vi "rename object.vi"(8 "error in":errorcluster, 9 "label_visible":bool, 10 "new_label_name":string, 11 "id":string) -> (0 "error out":errorcluster)   [LabVIEW 2020]
doc: "Renames an objects label.text property, can be a control/indicator or a block diagram element like a constant."
uses:
  G-AI Core/G-AI Core.lvlib
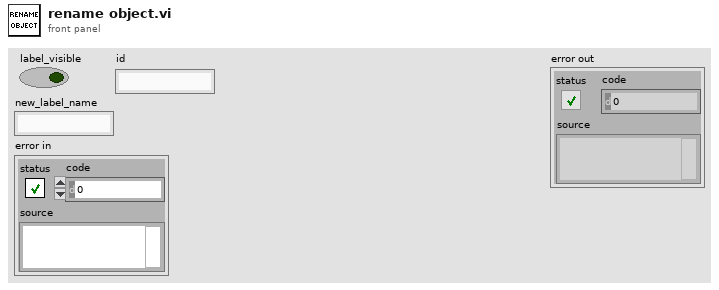
[diagram p1: front panel]
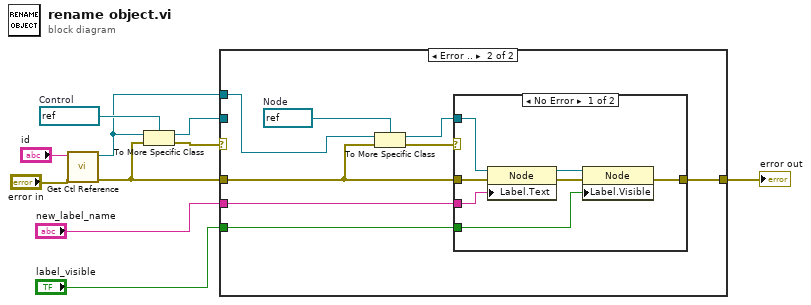
[diagram p0: block diagram]
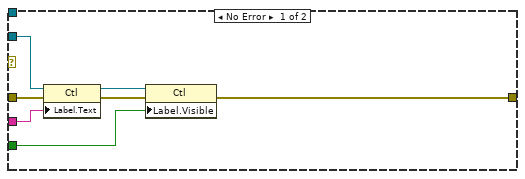
[diagram p2: hidden frame]
diagram:
  w9 = refnum<vi> refnum  # Control
  n1 = call "Get Ctl Reference.vi"("error in"="error in", "id"="id") -> ("error out"=w8:errorcluster, "ctl reference"=w7:refnum<vi>)  [unwired: 8 in]
  n2 = To More Specific Class(target class=w9, reference=w7, error in=w8) -> (specific class reference=w3:refnum<vi>, error out=w10:errorcluster)
  n3 = case shown="Error .." w10 {
    tunnel: w7 -> [_ w25]
    tunnel: "new_label_name" -> [w17 w19]
    tunnel: "label_visible" -> [w15 w20]
    tunnel: [w14 w23] -> w6
    tunnel: w8 -> [w12 w18]
    tunnel: w3 -> [w11 _]
    frame No Error {
      n4 = property class="Ctl"(reference=w11, error in=w12, "Label.Text"=w17) -> (reference out=w16:refnum<vi>, error out=w13:errorcluster)
      n5 = property class="Ctl"(reference=w16, error in=w13, "Label.Visible"=w15) -> (error out=w14:errorcluster)  [unwired: 1 out]
    }
    frame Error {
      w24 = refnum<vi> refnum  # Node
      n6 = To More Specific Class(target class=w24, reference=w25, error in=w18) -> (specific class reference=w21:refnum<vi>, error out=w22:errorcluster)
      n7 = case shown="No Error" w22 {
        tunnel: [w30 w33] -> w23
        tunnel: w21 -> [w31 _]
        tunnel: w20 -> [w28 _]
        tunnel: w19 -> [w27 _]
        tunnel: w18 -> [w26 w33]
        frame No Error {
          n8 = property class="Node"(reference=w31, error in=w26, "Label.Text"=w27) -> (reference out=w29:refnum<vi>, error out=w32:errorcluster)
          n9 = property class="Node"(reference=w29, error in=w32, "Label.Visible"=w28) -> (error out=w30:errorcluster)  [unwired: 1 out]
        }
        frame Error {
        }
      }
    }
  }
  "error out" <- w6
